vi "MonitorIndexCount.vi"(0 "Axis In":enum16{"X", "Y", "Z"}(ring), 11 "error in (no error)":errorcluster) -> (4 "Axis Out":T1, 6 "Index Count":u16, 15 "error out":errorcluster)   [LabVIEW 2009]
doc: "Batch count of index currently executing."
uses:
  typedefs/AxisSelect_Enum.ctl
  typedefs/Ultra3000/Func.ctl
  typedefs/Ultra3000/Cmds.ctl
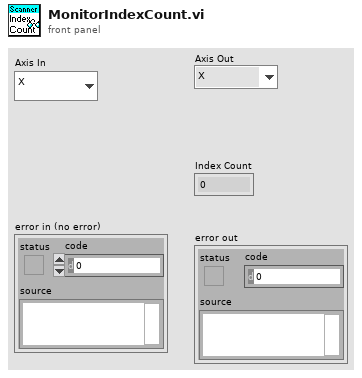
[diagram p1: front panel]
types:
  T1 = typedef "AxisSelect_Enum.ctl" = enum16{"X", "Y", "Z", "Axis Space"}
  T2 = typedef "Cmds.ctl" = u16
  T3 = typedef "Func.ctl" = u16
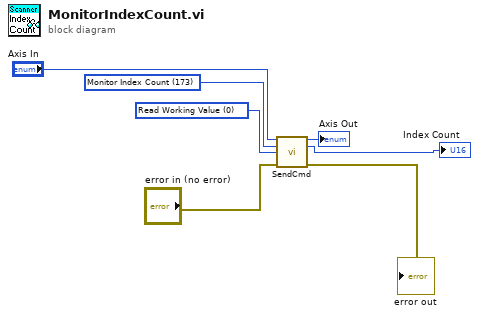
[diagram p0: block diagram]
diagram:
  w3 = T2 173 items=["Drive Status"=115, "Position Command"=128, "Run Status"=117, "Fault Status"=116, "Position Error"=129, "Auto-Start Homing"=196, "Start Homing"=205, "Homing Type"=197, "Monitor Index Count"=173, "Motor Position"=126, "Velocity Motor"=133, "Power-Up Status"=1, "Drive Name"=6, "Position Window Size"=22, "Position Window Time"=23, "Zero Speed Limit"=34, "Speed Window Size"=35, "Up to Speed Limit"=37, "Forward Current Limit"=47, "Reverse Current Limit"=48, "Override Mode"=67, "Operation Mode"=90, "Host Control Mode"=97, "Reset Drive"=106, "Drive Enable"=107, "Setpoint Current"=108, "Setpoint Velocity"=109, "Setpoint Acceleration"=110, "Reset Faults"=111, "Position Comparator"=349, "Postition Comparator Polarity"=350, "Position Rollover Enable"=404, "Baud Rate"=80, "Frame Format"=81, "Drive Address"=82, "Broadcast Address"=83, "Auto-start Indexing"=88, "Start Index"=112, "Host Index"=184, "Index Type"=174, "Index Dist/Pos"=175, "Index Reg Dist"=176, "Index Velocity"=177, "Index Acceleration"=178, "Index Deceleration"=179, "Index Dwell"=180, "Index Count"=181, "Index Termination"=182, "Index Pointer"=183, "Index Abort Deceleration"=185, "Positive Soft Pos Limit"=216, "Define Home"=113, "Negative Soft Pos Limit"=217] ("Command")
  w7 = T3 0 items=["Read Working Value", "Write Working Value", "Read Non-Volatile Value", "Write Non-Volatile and Woring Value", "Copy Non-Volatile Value to Working Value", "Copy Working Value to Non-Volatile Value", "Read Default Value", "Copy Default Value to Non-Volatile and Working Values", "Read Min Value", "Read Max Value", "Read Array Index Min", "Read Array Index Max"] ("Function")
  n1 = call "SendCmd.vi"("Axis In"="Axis In", "Command"=w3, "Function"=w7, "error in (no error)"="error in (no error)") -> ("Axis Out"=→"Axis Out":T1, "Data"=→"Index Count":i32, "error out"=→"error out":errorcluster)  [unwired: 8 in, 1 out]
